vi "Insert.vi"(11 "point":cluster{i64, i64, i64}) -> (3 "key already included?":bool)   [LabVIEW 2021, in "d18.lvlib"]
uses:
  d18.lvlib
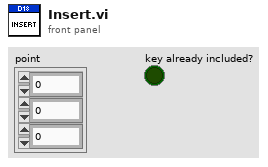
[diagram p1: front panel]
types:
  T1 = cluster{"point":cluster{i64, i64, i64}, "Response Notifier":refnum<notifier>}
  T2 = cluster{string, cluster{"point":cluster{i64, i64, i64}, "Response Notifier":refnum<notifier>}}
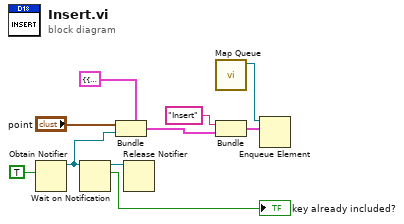
[diagram p0: block diagram]
diagram:
  n1 = Obtain Notifier(notification data type=TRUE ("key already included?")) -> (notifier out=w1:refnum<notifier>)  [unwired: 3 in, 2 out]
  n2 = Wait on Notification(notifier=w1) -> (notifier out=w9:refnum<notifier>, notification=→"key already included?":bool)  [unwired: 3 in, 2 out]
  n3 = Bundle(cluster=T1 {"point"={0, 0, 0}, "Response Notifier"=refnum}, "point"="point", "Response Notifier"=w1) -> (w8:T1)
  n4 = Release Notifier(notifier=w9) -> ()  [unwired: 2 in, 3 out]
  n5 = call "Map Queue.vi"() -> ("Queue out"=w5:refnum<queue>)  [unwired: 11 in]
  n6 = Bundle("Insert", w8) -> (w6:T2)  [unwired: 1 in]
  n7 = Enqueue Element(queue=w5, element=w6) -> ()  [unwired: 2 in, 3 out]
